vi "StartTrial.vi"(8 "error in (no error)":errorcluster, 11 "TrialBasedExperiment in":refnum<class "MouseBar.lvclass">) -> (0 "error out":errorcluster, 3 "TrialBasedExperiment out":refnum<class "MouseBar.lvclass">)   [LabVIEW 2011, in "MouseBar.lvclass"]
uses:
  MouseBar.lvclass
  Trial Based Experiment Statechart/PassiveExperiment/PassiveExperiment.lvclass
  Matlab API/Matlab API.lvlib
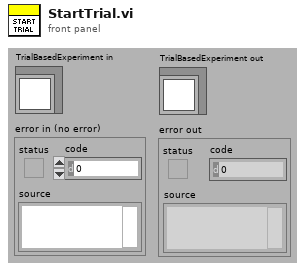
[diagram p1: front panel]
types:
  T1 = cluster{"Intertrial":dbl, "AcquireFixation":dbl, "HoldFixation":dbl, "DelayPeriod":dbl, "ResponsePeriod":dbl}
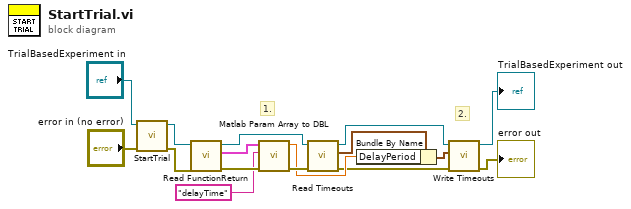
[diagram p0: block diagram]
diagram:
  # "2."
  # "1."
  n1 = call-parent "StartTrial.vi"("error in (no error)"="error in (no error)", "TrialBasedExperiment in"="TrialBasedExperiment in") -> ("error out"=w3:errorcluster, "TrialBasedExperiment out"=w4:refnum<class "MouseBar.lvclass">)  [unwired: 8 in]
  n2 = call-dynamic "Read FunctionReturn.vi"("error in (no error)"=w3, "MatlabExperiment in"=w4) -> ("error out"=w13:errorcluster, "FunctionReturn"=w8:cluster{"Name":string, "Data":variant}[], "MatlabExperiment out"=w5:refnum<class "MouseBar.lvclass">)  [unwired: 7 in]
  n3 = call "Matlab Param Array to DBL.vi"("error in (no error)"=w13, "Name"="delayTime", "Matlab Param Array"=w8) -> ("error out"=w14:errorcluster, "data"=w11:dbl)  [unwired: 7 in]
  n4 = call-dynamic "Read Timeouts.vi"("error in (no error)"=w14, "TrialBasedExperiment in"=w5) -> ("error out"=w7:errorcluster, "Timeouts"=w10:T1, "TrialBasedExperiment out"=w6:refnum<class "MouseBar.lvclass">)  [unwired: 7 in]
  n5 = Bundle By Name(cluster=w10, "DelayPeriod"=w11) -> (w12:T1)
  n6 = call-dynamic "Write Timeouts.vi"("error in (no error)"=w7, "Timeouts"=w12, "TrialBasedExperiment in"=w6) -> ("error out"=→"error out":errorcluster, "TrialBasedExperiment out"=→"TrialBasedExperiment out":refnum<class "MouseBar.lvclass">)  [unwired: 7 in]
